vi "mecanum 1.vi"() -> ()   [LabVIEW 2012, in "Mecanum Drive.lvrbt"]
uses:
  Mecanum Drive.lvrbt
  <vilib>/NXT/Hardware/Plugins/Tetrix DC Motor/TetrixDCMotorAddress.ctl
  <vilib>/FTC/FTC Calculate Drive Power - Arcade Right.vi
  <vilib>/FTC/FTC Calculate Drive Power - Arcade Left.vi
  <vilib>/NXT/NXTIO Xnodes/NXTIONodeSubVIs/TETRIX IO Move DC Motors.vi
  <vilib>/NXT/NXTIO Xnodes/NXTIONodeSubVIs/TETRIX IO Check Battery.vi
  <vilib>/NXT/NXTIO Xnodes/NXTIONodeSubVIs/TETRIX IO Stop DC Motors.vi
  <vilib>/NXT/NXTIO Xnodes/AddressXNode/NXTIOAddress.xnode
  <vilib>/NXT/Subs/LVHSConnector.ctl
  <vilib>/NXT/NXTIO Xnodes/NXTIOXNode/NXTIO.xnode
  <vilib>/NXT/LegoClasses/BrickReference/BrickReference.lvclass
panel:
  in  "Drive Power":i8=100 min=-100 max=100
  # "This VI was generated based on your configuration in the Remote Control Editor. You may modify the code as needed for your robot. To test this program for an FTC match, return to the Remote Control Editor, select the \"Run Program\" tab, and choose \"Teleop\"."
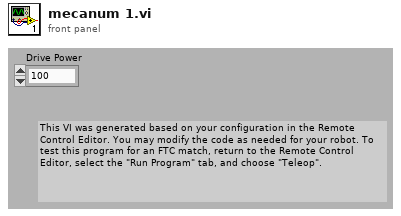
[diagram p1: front panel]
types:
  T1 = typedef "TetrixDCMotorAddress.ctl" = i32
  T2 = cluster{"TetrixDCMotor":T1, "TetrixDCMotor 2":T1}
  T3 = typedef "LVHSConnector.ctl" = refnum<class "BrickReference.lvclass">
  T4 = typedef "FTC ControllerState.ctl" = cluster{"Left X":i8, "Left Y":i8, "Right X":i8, "Right Y":i8, "Button Encoding 9-12":u8, "Button Encoding 1-8":u8, "POV":T5}
  T5 = typedef "FTC POVState.ctl" = i8
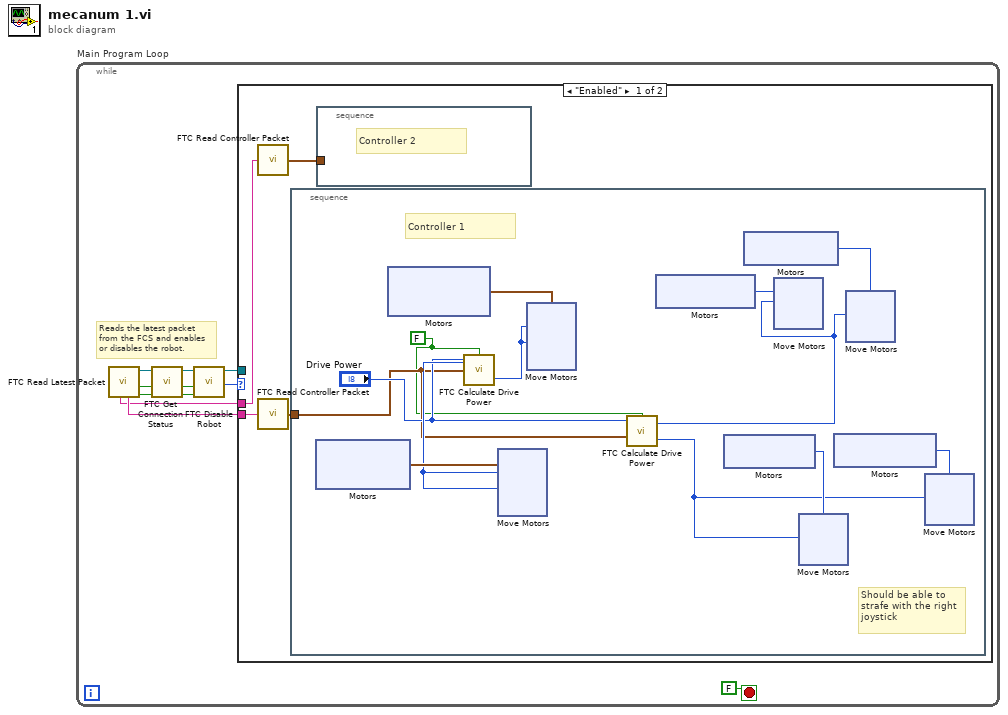
[diagram p0: block diagram]
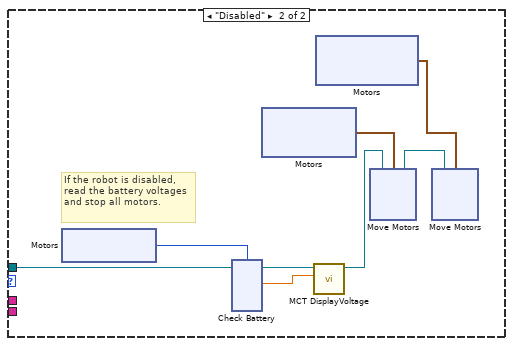
[diagram p2: hidden frame]
diagram:
  n1 = while "Main Program Loop" {
    stop <- FALSE stop-if-true
    # "Reads the latest packet\nfrom the FCS and enables\nor disables the robot."
    n2 = call <vilib>:"FTC Read Latest Packet.vi"() -> ("Packet Received?"=w8:bool, "Stopped?"=w5:bool, "NXT/EV3"=w7:T3, "Controller 1"=w10:string, "Controller 2"=w9:string)  [unwired: 6 in, 1 out]
    n3 = call <vilib>:"FTC Get Connection Status.vi"("Packet Received?"=w8, "Stopped?"=w5, "NXT/EV3"=w7) -> ("Online?"=w2:bool, "Stopped?"=w3:bool, "NXT/EV3"=w4:T3)  [unwired: 5 in]
    n4 = call <vilib>:"FTC Disable Robot.vi"("Online?"=w2, "Stopped?"=w3, "NXT/EV3"=w4) -> ("Enabled?"=w6:enum16{"Disabled", "Enabled"}, "NXT/EV3"=w1:T3)  [unwired: 3 in]
    n5 = case "disableCase" shown="\"Enabled\"" w6 {
      tunnel: w10 -> [w15 _]
      tunnel: w9 -> [w14 _]
      tunnel: w1 -> [_ w86]
      frame "Enabled" {
        n6 = call <vilib>:"FTC Read Controller Packet.vi"("Packet"=w14) -> ("Controller State"=w12:T4)  [unwired: 4 in]
        n7 = call <vilib>:"FTC Read Controller Packet.vi"("Packet"=w15) -> ("Controller State"=w13:T4)  [unwired: 4 in]
        n8 = stacked-sequence "controller1Actions" {
          tunnel: w13 -> [w23]
          frame #0 {
            w21 = FALSE ("Reverse")
            # "Should be able to\nstrafe with the right\njoystick"
            # "Controller 1"
            n9 = xnode ("Motors")() -> ("Motor"=w27:cluster{"TetrixDCMotor":T1, "TetrixDCMotor":T1})
            n10 = xnode ("Motors")() -> ("Motor"=w28:cluster{"TetrixDCMotor":T1, "TetrixDCMotor":T1})
            n11 = call-poly <vilib>:"FTC Calculate Drive Power.vi"("Reverse"=w21, "Controller State"=w23, "Power Level (50)"="Drive Power") -> ("Right Motor Power"=w26:i8, "Left Motor Power"=w25:i8)  [unwired: 1 in]
            n12 = xnode ("Move Motors")("Power/Speed 2"=w25, "Power/Speed 1"=w25, "Motors"=w27) -> ()  [unwired: 1 in, 1 out]
            n13 = xnode ("Move Motors")("Power/Speed 2"=w26, "Power/Speed 1"=w26, "Motors"=w28) -> ()  [unwired: 1 in, 1 out]
            n14 = call-poly <vilib>:"FTC Calculate Drive Power.vi"("Reverse"=w21, "Controller State"=w23, "Power Level (50)"="Drive Power") -> ("Right Motor Power"=w18:i8, "Left Motor Power"=w17:i8)  [unwired: 1 in]
            n15 = xnode ("Motors")() -> ("Motor"=w19:T1)
            n16 = xnode ("Motors")() -> ("Motor"=w20:T1)
            n17 = xnode ("Motors")() -> ("Motor"=w22:T1)
            n18 = xnode ("Move Motors")("Power/Speed 1"=w17, "Motors"=w19) -> ()  [unwired: 1 in, 1 out]
            n19 = xnode ("Move Motors")("Power/Speed 1"=w18, "Motors"=w20) -> ()  [unwired: 1 in, 1 out]
            n20 = xnode ("Motors")() -> ("Motor"=w16:T1)
            n21 = xnode ("Move Motors")("Power/Speed 1"=w17, "Motors"=w22) -> ()  [unwired: 1 in, 1 out]
            n22 = xnode ("Move Motors")("Power/Speed 1"=w18, "Motors"=w16) -> ()  [unwired: 1 in, 1 out]
          }
        }
        n23 = stacked-sequence "controller2Actions" {
          tunnel: w12 -> [_]
          frame #0 {
            # "Controller 2"
          }
        }
      }
      frame "Disabled" {
        # "If the robot is disabled, read the battery voltages and stop all motors."
        n24 = xnode ("Motors")() -> ("Motor"=w85:T1)
        n25 = xnode ("Check Battery")("Motors"=w85, "NXT/EV3"=w86) -> ("Voltage 1"=w84:sgl, "NXT/EV3"=w83:T3)
        n26 = xnode "Motors"() -> ("Motor"=w82:cluster{"TetrixDCMotor":T1, "TetrixDCMotor":T1})
        n27 = call <vilib>:"MCT DisplayVoltage.vi"("Motor Voltage"=w84, "NXT/EV3"=w83) -> ("NXT/EV3"=w81:T3)  [unwired: 9 in]
        n28 = xnode "Motors"() -> ("Motor"=w80:cluster{"TetrixDCMotor":T1, "TetrixDCMotor":T1})
        n29 = xnode "Move Motors"("Motors"=w82, "NXT/EV3"=w81) -> ("NXT/EV3"=w79:T3)
        n30 = xnode "Move Motors"("Motors"=w80, "NXT/EV3"=w79) -> ()  [unwired: 1 out]
      }
    }
  }
